vi "Transform Table with merge cells.vi"(0 "Titles and Datas 2D [ ] IN":string[][](array[string]), 7 "Row  [ ]":T1, 11 "error in (no error)":errorcluster) -> (4 "Titles and Datas 2D [ ] OUT":string[][](array[string]), 15 "error duplicate":errorcluster)   [LabVIEW 2020, in "Exaprom PDF.lvlib"]
doc: "Version 2.0\nDeveloped by Jean-Marc Simard\nCopyright © 2013, Exaprom Inc.\nAll rights reserved.\nLicense: BSD\n\nWith iTextSharp 4.1.6 (http://itextsharp.sourceforge.net)\nunder Mozilla Public License Version 1.1\n(http://www.mozilla.org/MPL/MPL-1.1.html)"
uses:
  <userlib>/labview-PDF-writer-master/Exaprom PDF.lvlib
  <userlib>/labview-PDF-writer-master/Controls/Table Controls/Table Appearance and Font Row [ ].ctl
  <userlib>/labview-PDF-writer-master/Controls/Table Controls/One Row Appearance.ctl
  <userlib>/labview-PDF-writer-master/Controls/Table Controls/Row from to.ctl
  <userlib>/labview-PDF-writer-master/Controls/Table Controls/Cell, Alignment, LS and Font - hide Vmerge.ctl
  <userlib>/labview-PDF-writer-master/Controls/Table Controls/Cell Type, Alignment and LS.ctl
  <userlib>/labview-PDF-writer-master/Controls/Table Controls/Cell Alignment 20px.ctl
  <userlib>/labview-PDF-writer-master/Controls/Table Controls/Text vertical arrangement.ctl
  <userlib>/labview-PDF-writer-master/Controls/Text Controls/Line spacing.ctl
  <userlib>/labview-PDF-writer-master/Controls/Table Controls/Cell Appearance.ctl
  <userlib>/labview-PDF-writer-master/Controls/Table Controls/Cell Border 20 px.ctl
  <userlib>/labview-PDF-writer-master/Controls/Table Controls/Merge Horizontal.ctl
  <userlib>/labview-PDF-writer-master/Controls/Table Controls/Merge Vertical.ctl
  <userlib>/labview-PDF-writer-master/Controls/Font Controls/Font complete cluster.ctl
  <userlib>/labview-PDF-writer-master/Controls/Font Controls/Font size.ctl
  <userlib>/labview-PDF-writer-master/Controls/Font Controls/Font color.ctl
  <userlib>/labview-PDF-writer-master/Controls/Font Controls/Type and encoding.ctl
  <userlib>/labview-PDF-writer-master/Controls/Text Controls/Unicode/Type and run direction.ctl
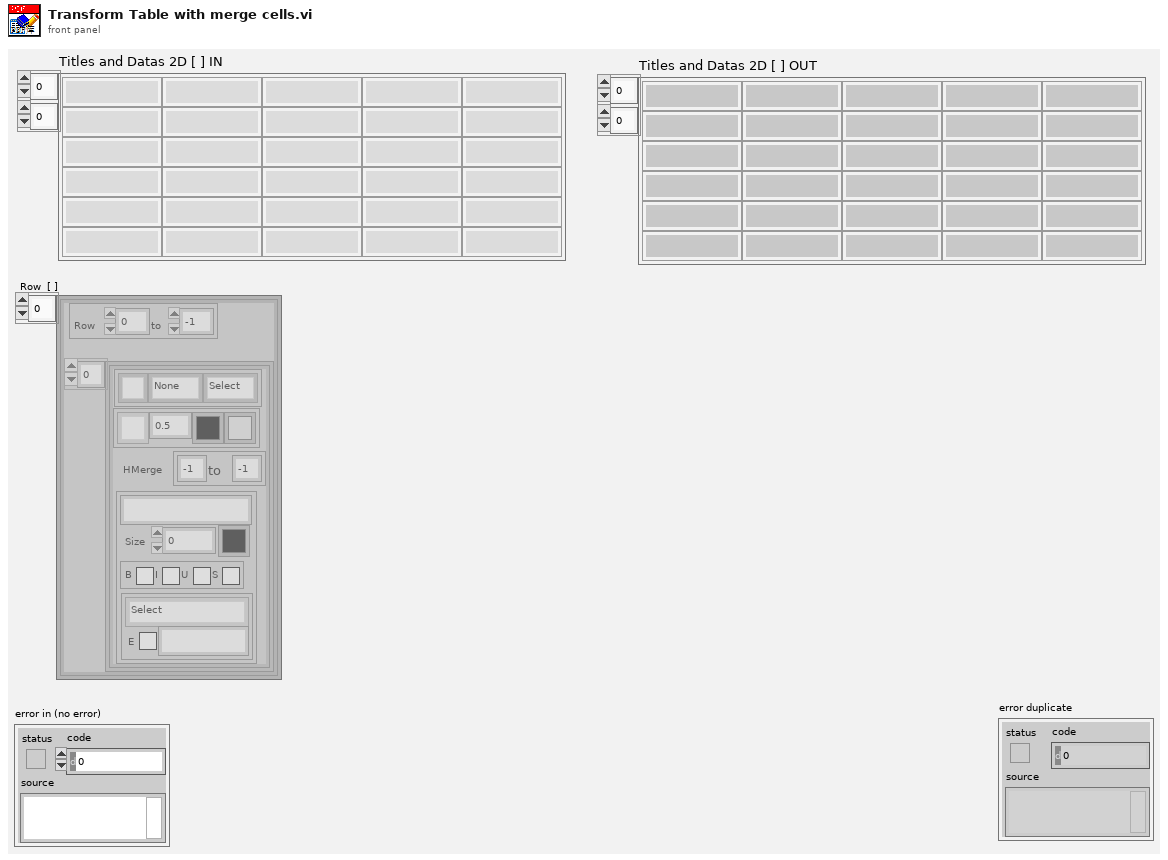
[diagram p1: front panel]
types:
  T1 = typedef "Exaprom PDF.lvlib/Table Appearance and Font Row [ ].ctl" = T2[]
  T2 = typedef "Exaprom PDF.lvlib/One Row Appearance.ctl" = cluster{"Row":T3, "Cell [ ]":T4[]}
  T3 = typedef "Exaprom PDF.lvlib/Row from to.ctl" = cluster{"From #":i16, "to #":i16}
  T4 = typedef "Exaprom PDF.lvlib/Cell, Alignment, LS and Font - hide Vmerge.ctl" = cluster{"Text":T5, "Cell Appearance":T9, "HMerge":T11, "VMerge":T12, "Font":T13}
  T5 = typedef "Exaprom PDF.lvlib/Cell Type, Alignment and LS.ctl" = cluster{"Cell Alignment":T6, "Text rotation":T7, "Line spacing":T8}
  T6 = typedef "Exaprom PDF.lvlib/Cell Alignment 20px.ctl" = u16
  T7 = typedef "Exaprom PDF.lvlib/Text vertical arrangement.ctl" = enum16{"None", "Clockwise", "Counterclockwise"}
  T8 = typedef "Exaprom PDF.lvlib/Line spacing.ctl" = enum16{"Select", "1.0", "1.5", "2.0"}
  T9 = typedef "Exaprom PDF.lvlib/Cell Appearance.ctl" = cluster{"Border":T10, "Thickness":sgl, "Color":u32, "BG":u32}
  T10 = typedef "Exaprom PDF.lvlib/Cell Border 20 px.ctl" = u16
  T11 = typedef "Exaprom PDF.lvlib/Merge Horizontal.ctl" = cluster{"From":i8, "to":i8}
  T12 = typedef "Exaprom PDF.lvlib/Merge Vertical.ctl" = cluster{"From":i8, "to":i8}
  T13 = typedef "Exaprom PDF.lvlib/Font complete cluster.ctl" = cluster{"Name":string, "Size":T14, "Color":T15, "Style":cluster{"Bold":bool, "Italic":bool, "Underline":bool, "Strikeout":bool}, "Type":T16}
  T14 = typedef "Exaprom PDF.lvlib/Font size.ctl" = sgl
  T15 = typedef "Exaprom PDF.lvlib/Font color.ctl" = u32
  T16 = typedef "Exaprom PDF.lvlib/Type and encoding.ctl" = cluster{"Type&direction":T17, "Embedded":bool, "Encoding":string}
  T17 = typedef "Exaprom PDF.lvlib/Type and run direction.ctl" = enum16{"Select", "ASCII", "UTF-16", "UTF-16 (default)", "UTF-16 (LTR)", "UTF-16 (RTL)"}
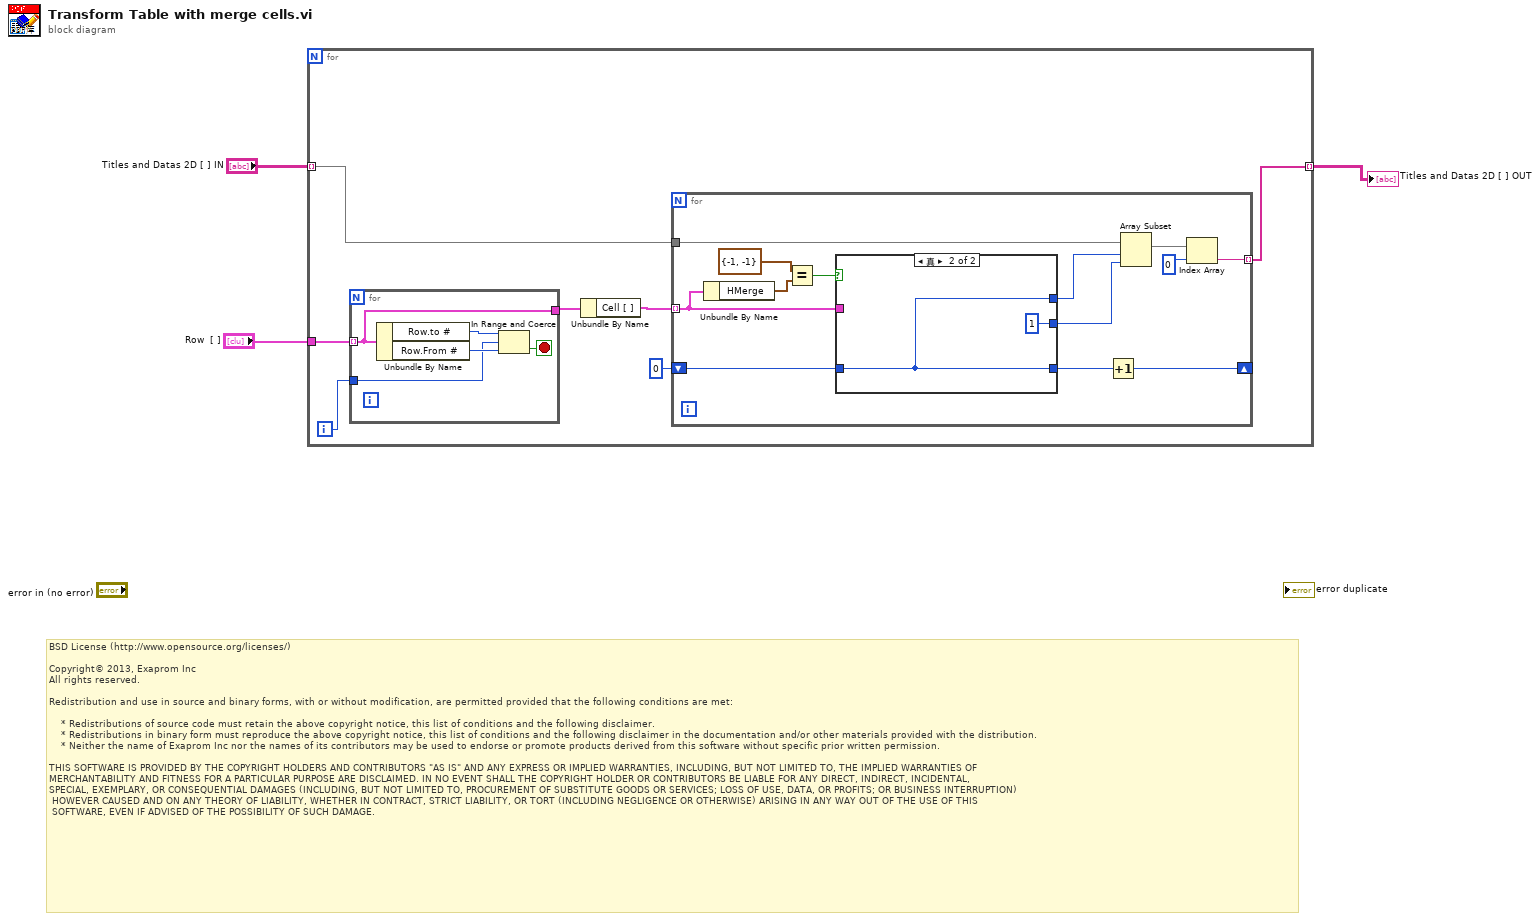
[diagram p0: block diagram]
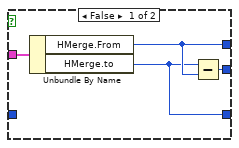
[diagram p2: hidden frame]
diagram:
  # "BSD License (http://www.opensource.org/licenses/)\n\nCopyright© 2013, Exaprom Inc\nAll rights reserved.\n\nRedistribution and use in source and binary forms, with or without modification, are permitted provided that the following conditions are met:\n\n    * Redistributions of source code must retain the above copyright notice, this list of conditions and the following disclaimer.\n    * Redistributions in binary form must reproduce the above copyright notice, this list of conditions and the following disclaimer in the documentation and/or other materials provided with the distribution.\n    * Neither the name of Exaprom Inc nor the names of its contributors may be used to endorse or promote products derived from this software without specific prior written permission.\n\nTHIS SOFTWARE IS PROVIDED BY THE COPYRIGHT HOLDERS AND CONTRIBUTORS \"AS IS\" AND ANY EXPRESS OR IMPLIED WARRANTIES, INCLUDING, BUT NOT LIMITED TO, THE IMPLIED WARRANTIES OF \nMERCHANTABILITY AND FITNESS FOR A PARTICULAR PURPOSE ARE DISCLAIMED. IN NO EVENT SHALL THE COPYRIGHT HOLDER OR CONTRIBUTORS BE LIABLE FOR ANY DIRECT, INDIRECT, INCIDENTAL,\nSPECIAL, EXEMPLARY, OR CONSEQUENTIAL DAMAGES (INCLUDING, BUT NOT LIMITED TO, PROCUREMENT OF SUBSTITUTE GOODS OR SERVICES; LOSS OF USE, DATA, OR PROFITS; OR BUSINESS INTERRUPTION)\n HOWEVER CAUSED AND ON ANY THEORY OF LIABILITY, WHETHER IN CONTRACT, STRICT LIABILITY, OR TORT (INCLUDING NEGLIGENCE OR OTHERWISE) ARISING IN ANY WAY OUT OF THE USE OF THIS\n SOFTWARE, EVEN IF ADVISED OF THE POSSIBILITY OF SUCH DAMAGE."
  n1 = for {
    tunnel: [w5] -> w3 mode=indexing
    tunnel: "Titles and Datas 2D [ ] IN" -> [w6] mode=indexing
    tunnel: "Row  [ ]" -> [w10]
    i -> [w4]
    n2 = for {
      tunnel: w10 -> [w31] mode=indexing
      tunnel: [w31] -> w9
      tunnel: w4 -> [w30]
      stop <- w32 stop-if-true
      n3 = Unbundle By Name(w31) -> ("Row.to #"=w34:i16, "Row.From #"=w33:i16)
      n4 = In Range and Coerce(upper limit=w34, x=w30, lower limit=w33) -> (In Range?=w32:bool)  [unwired: 1 out]
    }
    n5 = Unbundle By Name(w9) -> ("Cell [ ]"=w8:T4[])
    n6 = for {
      tunnel: w8 -> [w15] mode=indexing
      tunnel: w6 -> [w23]
      tunnel: [w18] -> w5 mode=indexing
      shift-right: [w16] -> _
      shift-left: 0 -> [w11]
      n7 = Unbundle By Name(w15) -> ("HMerge"=w14:T11)
      n8 = Equal?(x=T11 {"From"=-1, "to"=-1}, y=w14) -> (x = y?=w12:bool)
      n9 = case shown="真" w12 {
        tunnel: [w27 w29] -> w22
        tunnel: [w26 i8 1] -> w21
        tunnel: [w25 w29] -> w17
        tunnel: w15 -> [w24 _]
        tunnel: w11 -> [_ w29]
        frame False {
          n10 = Unbundle By Name(w24) -> ("HMerge.From"=w27:i8, "HMerge.to"=w25:i8)
          n11 = Subtract(x=w25, y=w27) -> (x-y=w26:i8)
        }
        frame True {
        }
      }
      n12 = Increment(x=w17) -> (x+1=w16:i32)
      n13 = Array Subset(array=w23, index=w22, length=w21) -> (w20:string[])
      n14 = Index Array(array=w20, index=0) -> (element=w18:string)
    }
  }
  "Titles and Datas 2D [ ] OUT" <- w3
